vi "Get data product.vi"(8 "error in (no error)":errorcluster, 9 "Credito":dbl, 10 "Selector":dbl, 11 "Paquetes Disonibles in":refnum<class "Paquetes Disonibles.lvclass">) -> (0 "error out":errorcluster, 3 "Paquetes Disonibles out":refnum<class "Paquetes Disonibles.lvclass">)   [LabVIEW 2021, in "Paquetes Disonibles.lvlib" / "Paquetes Disonibles.lvclass"]
uses:
  Paquetes Disonibles.lvclass
  C:/Program Files (x86)/National Instruments/LabVIEW 2021/vi.lib/ActorFramework/Actor/Actor.lvclass
  Paquetes Disonibles.lvclass/Paquetes Disonibles.ctl
  <vilib>/ActorFramework/Actor/Actor.lvclass/Actor.ctl
  User Interface Messages/Get Change Msg/Get Change Msg.lvclass/Get Change Msg.ctl
  <vilib>/ActorFramework/Message Enqueuer/Message Enqueuer.lvclass/Message Enqueuer.ctl
  User Interface Messages/Get Product Msg/Get Product Msg.lvclass/Get Product Msg.ctl
  <vilib>/ActorFramework/Message Enqueuer/Enqueue.vi
  User Interface Messages/Get Change Msg/Get Change Msg.lvclass
  C:/Program Files (x86)/National Instruments/LabVIEW 2021/vi.lib/ActorFramework/Message/Message.lvclass
  User Interface Messages/Get Product Msg/Get Product Msg.lvclass
  <vilib>/ActorFramework/Message Priority Queue/Priority Enqueue.vi
  <vilib>/ActorFramework/Actor/Actor.lvclass
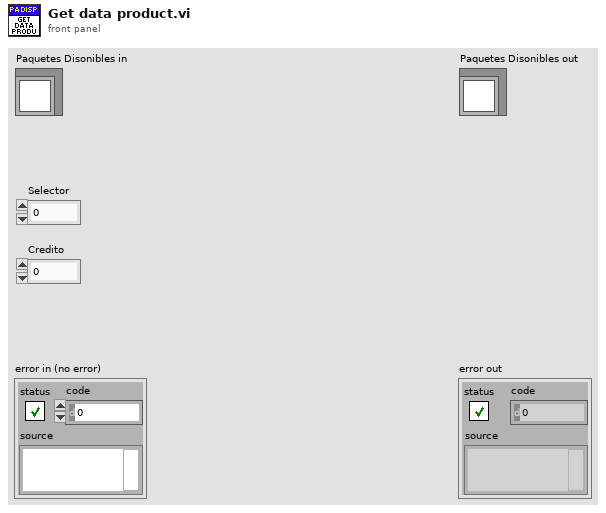
[diagram p1: front panel]
types:
  T1 = cluster{"Products":cluster{"Name":string, "Cost":u8, "Inventory":dbl}, "Products 2":cluster{"Name":string, "Cost":u8, "Inventory":dbl}, "Products 3":cluster{"Name":string, "Cost":u8, "Inventory":dbl}, "Products 4":cluster{"Name":string, "Cost":u8, "Inventory":dbl}, "Products 5":cluster{"Name":string, "Cost":u8, "Inventory":dbl}}
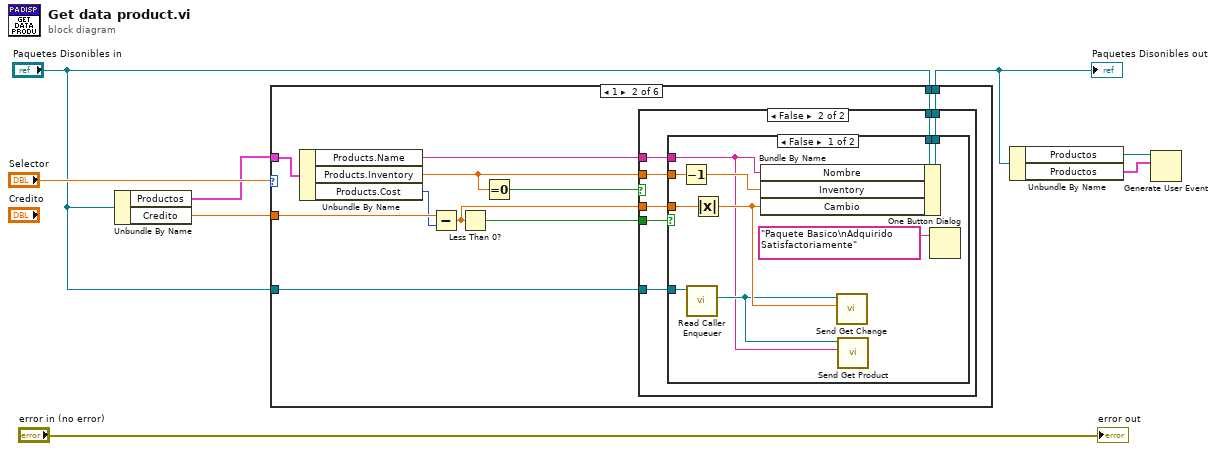
[diagram p0: block diagram]
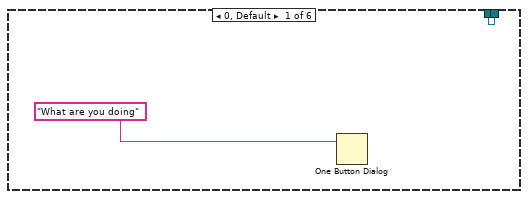
[diagram p2: hidden frame]
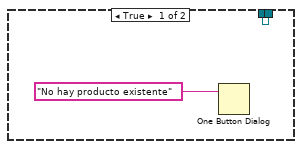
[diagram p3: hidden frame]
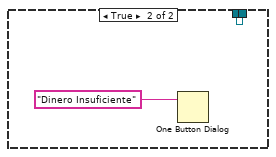
[diagram p4: hidden frame]
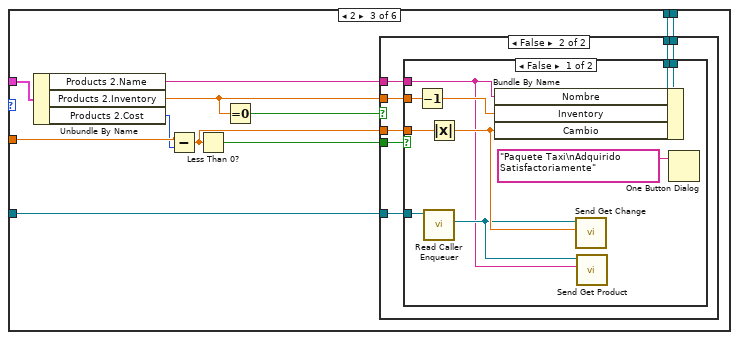
[diagram p5: hidden frame]
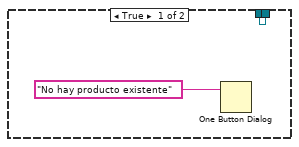
[diagram p6: hidden frame]
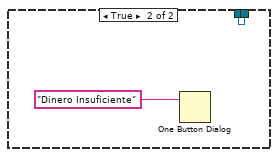
[diagram p7: hidden frame]
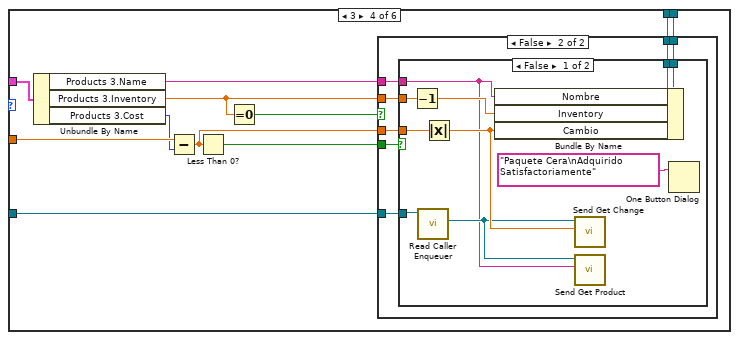
[diagram p8: hidden frame]
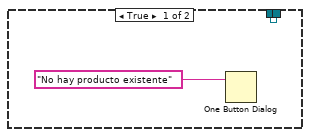
[diagram p9: hidden frame]
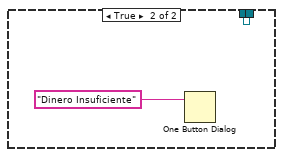
[diagram p10: hidden frame]
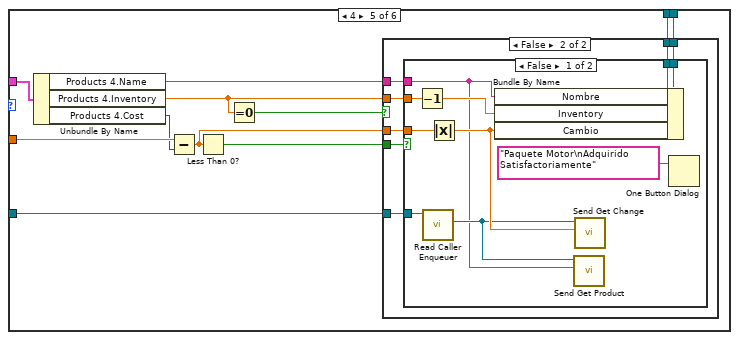
[diagram p11: hidden frame]
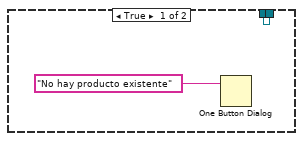
[diagram p12: hidden frame]
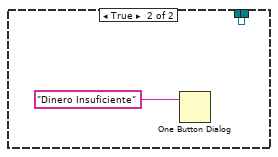
[diagram p13: hidden frame]
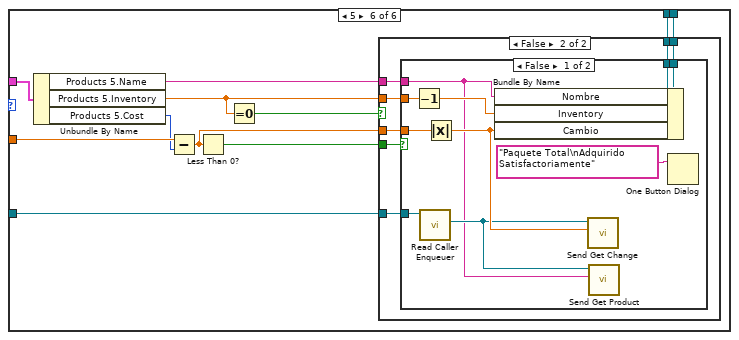
[diagram p14: hidden frame]
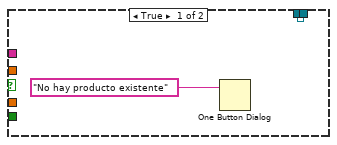
[diagram p15: hidden frame]
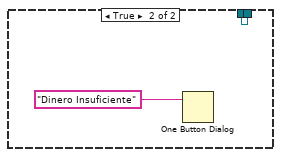
[diagram p16: hidden frame]
diagram:
  n1 = Unbundle By Name("Paquetes Disonibles in") -> ("Productos"=w6:T1, "Credito"=w2:dbl)
  n2 = case shown="1" "Selector" {
    tunnel: w2 -> [_ w15 w47 w79 w111 w143]
    tunnel: w6 -> [_ w21 w53 w85 w117 w149]
    tunnel: "Paquetes Disonibles in" -> [w10 w18 w50 w82 w114 w146]
    tunnel: [w10 w17 w49 w81 w113 w145] -> w5
    tunnel: "Paquetes Disonibles in" -> [_ w11 w43 w75 w107 w139]
    frame 0, Default {
      n3 = One Button Dialog(message="What are you doing") -> ()  [unwired: 1 in, 1 out]
    }
    frame 1 {
      n4 = Unbundle By Name(w21) -> ("Products.Name"=w19:string, "Products.Inventory"=w12:dbl, "Products.Cost"=w14:u8)
      n5 = Subtract(x=w15, y=w14) -> (x-y=w16:dbl)
      n6 = Less Than 0?(x=w16) -> (x < 0?=w20:bool)
      n7 = Equal To 0?(x=w12) -> (x = 0?=w13:bool)
      n8 = case shown="False" w13 {
        tunnel: w20 -> [_ w30]
        tunnel: w12 -> [_ w29]
        tunnel: w19 -> [_ w28]
        tunnel: w18 -> [w22 w27]
        tunnel: [w22 w26] -> w17
        tunnel: w16 -> [_ w25]
        tunnel: w11 -> [_ w24]
        frame True {
          n9 = One Button Dialog(message="No hay producto existente") -> ()  [unwired: 1 in, 1 out]
        }
        frame False {
          n10 = case shown="False" w30 {
            tunnel: w29 -> [w40 _]
            tunnel: w28 -> [w31 _]
            tunnel: w27 -> [w39 w41]
            tunnel: [w38 w41] -> w26
            tunnel: w25 -> [w36 _]
            tunnel: w24 -> [w34 _]
            frame False {
              n11 = Decrement(x=w40) -> (x-1=w37:dbl)
              n12 = call <vilib>:"Read Caller Enqueuer.vi"("Actor"=w34) -> ("Caller Enqueuer"=w32:refnum<class "Message Enqueuer.lvclass">)  [unwired: 10 in]
              n13 = Absolute Value(x=w36) -> (abs(x)=w33:dbl)
              n14 = Bundle By Name(cluster=w39, "Nombre"=w31, "Inventory"=w37, "Cambio"=w33) -> (w38:refnum<class "Paquetes Disonibles.lvclass">)
              n15 = call "Send Get Change.vi"("Cambio"=w33, "Message Enqueuer"=w32) -> ()  [unwired: 8 in, 2 out]
              n16 = call "Send Get Product.vi"("Producto"=w31, "Message Enqueuer"=w32) -> ()  [unwired: 8 in, 2 out]
              n17 = One Button Dialog(message="Paquete Basico\nAdquirido Satisfactoriamente") -> ()  [unwired: 1 in, 1 out]
            }
            frame True {
              n18 = One Button Dialog(message="Dinero Insuficiente") -> ()  [unwired: 1 in, 1 out]
            }
          }
        }
      }
    }
    frame 2 {
      n19 = Unbundle By Name(w53) -> ("Products 2.Name"=w51:string, "Products 2.Inventory"=w44:dbl, "Products 2.Cost"=w46:u8)
      n20 = Subtract(x=w47, y=w46) -> (x-y=w48:dbl)
      n21 = Less Than 0?(x=w48) -> (x < 0?=w52:bool)
      n22 = Equal To 0?(x=w44) -> (x = 0?=w45:bool)
      n23 = case shown="False" w45 {
        tunnel: w52 -> [_ w62]
        tunnel: w44 -> [_ w61]
        tunnel: w51 -> [_ w60]
        tunnel: w50 -> [w55 w59]
        tunnel: [w55 w58] -> w49
        tunnel: w48 -> [_ w57]
        tunnel: w43 -> [_ w56]
        frame True {
          n24 = One Button Dialog(message="No hay producto existente") -> ()  [unwired: 1 in, 1 out]
        }
        frame False {
          n25 = case shown="False" w62 {
            tunnel: w61 -> [w72 _]
            tunnel: w60 -> [w63 _]
            tunnel: w59 -> [w71 w73]
            tunnel: [w70 w73] -> w58
            tunnel: w57 -> [w68 _]
            tunnel: w56 -> [w66 _]
            frame False {
              n26 = Decrement(x=w72) -> (x-1=w69:dbl)
              n27 = call <vilib>:"Read Caller Enqueuer.vi"("Actor"=w66) -> ("Caller Enqueuer"=w64:refnum<class "Message Enqueuer.lvclass">)  [unwired: 10 in]
              n28 = Absolute Value(x=w68) -> (abs(x)=w65:dbl)
              n29 = Bundle By Name(cluster=w71, "Nombre"=w63, "Inventory"=w69, "Cambio"=w65) -> (w70:refnum<class "Paquetes Disonibles.lvclass">)
              n30 = call "Send Get Change.vi"("Cambio"=w65, "Message Enqueuer"=w64) -> ()  [unwired: 8 in, 2 out]
              n31 = call "Send Get Product.vi"("Producto"=w63, "Message Enqueuer"=w64) -> ()  [unwired: 8 in, 2 out]
              n32 = One Button Dialog(message="Paquete Taxi\nAdquirido Satisfactoriamente") -> ()  [unwired: 1 in, 1 out]
            }
            frame True {
              n33 = One Button Dialog(message="Dinero Insuficiente") -> ()  [unwired: 1 in, 1 out]
            }
          }
        }
      }
    }
    frame 3 {
      n34 = Unbundle By Name(w85) -> ("Products 3.Name"=w83:string, "Products 3.Inventory"=w76:dbl, "Products 3.Cost"=w78:u8)
      n35 = Subtract(x=w79, y=w78) -> (x-y=w80:dbl)
      n36 = Less Than 0?(x=w80) -> (x < 0?=w84:bool)
      n37 = Equal To 0?(x=w76) -> (x = 0?=w77:bool)
      n38 = case shown="False" w77 {
        tunnel: w84 -> [_ w94]
        tunnel: w76 -> [_ w93]
        tunnel: w83 -> [_ w92]
        tunnel: w82 -> [w87 w91]
        tunnel: [w87 w90] -> w81
        tunnel: w80 -> [_ w89]
        tunnel: w75 -> [_ w88]
        frame True {
          n39 = One Button Dialog(message="No hay producto existente") -> ()  [unwired: 1 in, 1 out]
        }
        frame False {
          n40 = case shown="False" w94 {
            tunnel: w93 -> [w104 _]
            tunnel: w92 -> [w95 _]
            tunnel: w91 -> [w103 w105]
            tunnel: [w102 w105] -> w90
            tunnel: w89 -> [w100 _]
            tunnel: w88 -> [w98 _]
            frame False {
              n41 = Decrement(x=w104) -> (x-1=w101:dbl)
              n42 = call <vilib>:"Read Caller Enqueuer.vi"("Actor"=w98) -> ("Caller Enqueuer"=w96:refnum<class "Message Enqueuer.lvclass">)  [unwired: 10 in]
              n43 = Absolute Value(x=w100) -> (abs(x)=w97:dbl)
              n44 = Bundle By Name(cluster=w103, "Nombre"=w95, "Inventory"=w101, "Cambio"=w97) -> (w102:refnum<class "Paquetes Disonibles.lvclass">)
              n45 = call "Send Get Change.vi"("Cambio"=w97, "Message Enqueuer"=w96) -> ()  [unwired: 8 in, 2 out]
              n46 = call "Send Get Product.vi"("Producto"=w95, "Message Enqueuer"=w96) -> ()  [unwired: 8 in, 2 out]
              n47 = One Button Dialog(message="Paquete Cera\nAdquirido Satisfactoriamente") -> ()  [unwired: 1 in, 1 out]
            }
            frame True {
              n48 = One Button Dialog(message="Dinero Insuficiente") -> ()  [unwired: 1 in, 1 out]
            }
          }
        }
      }
    }
    frame 4 {
      n49 = Unbundle By Name(w117) -> ("Products 4.Name"=w115:string, "Products 4.Inventory"=w108:dbl, "Products 4.Cost"=w110:u8)
      n50 = Subtract(x=w111, y=w110) -> (x-y=w112:dbl)
      n51 = Less Than 0?(x=w112) -> (x < 0?=w116:bool)
      n52 = Equal To 0?(x=w108) -> (x = 0?=w109:bool)
      n53 = case shown="False" w109 {
        tunnel: w116 -> [_ w126]
        tunnel: w108 -> [_ w125]
        tunnel: w115 -> [_ w124]
        tunnel: w114 -> [w118 w123]
        tunnel: [w118 w122] -> w113
        tunnel: w112 -> [_ w121]
        tunnel: w107 -> [_ w120]
        frame True {
          n54 = One Button Dialog(message="No hay producto existente") -> ()  [unwired: 1 in, 1 out]
        }
        frame False {
          n55 = case shown="False" w126 {
            tunnel: w125 -> [w136 _]
            tunnel: w124 -> [w127 _]
            tunnel: w123 -> [w135 w137]
            tunnel: [w134 w137] -> w122
            tunnel: w121 -> [w132 _]
            tunnel: w120 -> [w129 _]
            frame False {
              n56 = Decrement(x=w136) -> (x-1=w133:dbl)
              n57 = call <vilib>:"Read Caller Enqueuer.vi"("Actor"=w129) -> ("Caller Enqueuer"=w128:refnum<class "Message Enqueuer.lvclass">)  [unwired: 10 in]
              n58 = Absolute Value(x=w132) -> (abs(x)=w130:dbl)
              n59 = Bundle By Name(cluster=w135, "Nombre"=w127, "Inventory"=w133, "Cambio"=w130) -> (w134:refnum<class "Paquetes Disonibles.lvclass">)
              n60 = call "Send Get Product.vi"("Producto"=w127, "Message Enqueuer"=w128) -> ()  [unwired: 8 in, 2 out]
              n61 = call "Send Get Change.vi"("Cambio"=w130, "Message Enqueuer"=w128) -> ()  [unwired: 8 in, 2 out]
              n62 = One Button Dialog(message="Paquete Motor\nAdquirido Satisfactoriamente") -> ()  [unwired: 1 in, 1 out]
            }
            frame True {
              n63 = One Button Dialog(message="Dinero Insuficiente") -> ()  [unwired: 1 in, 1 out]
            }
          }
        }
      }
    }
    frame 5 {
      n64 = Unbundle By Name(w149) -> ("Products 5.Name"=w147:string, "Products 5.Inventory"=w140:dbl, "Products 5.Cost"=w142:u8)
      n65 = Subtract(x=w143, y=w142) -> (x-y=w144:dbl)
      n66 = Less Than 0?(x=w144) -> (x < 0?=w148:bool)
      n67 = Equal To 0?(x=w140) -> (x = 0?=w141:bool)
      n68 = case shown="False" w141 {
        tunnel: w148 -> [_ w158]
        tunnel: w140 -> [_ w157]
        tunnel: w147 -> [_ w156]
        tunnel: w146 -> [w150 w155]
        tunnel: [w150 w154] -> w145
        tunnel: w144 -> [_ w153]
        tunnel: w139 -> [_ w152]
        frame True {
          n69 = One Button Dialog(message="No hay producto existente") -> ()  [unwired: 1 in, 1 out]
        }
        frame False {
          n70 = case shown="False" w158 {
            tunnel: w157 -> [w168 _]
            tunnel: w156 -> [w159 _]
            tunnel: w155 -> [w167 w169]
            tunnel: [w166 w169] -> w154
            tunnel: w153 -> [w164 _]
            tunnel: w152 -> [w162 _]
            frame False {
              n71 = Decrement(x=w168) -> (x-1=w165:dbl)
              n72 = call <vilib>:"Read Caller Enqueuer.vi"("Actor"=w162) -> ("Caller Enqueuer"=w160:refnum<class "Message Enqueuer.lvclass">)  [unwired: 10 in]
              n73 = Absolute Value(x=w164) -> (abs(x)=w161:dbl)
              n74 = Bundle By Name(cluster=w167, "Nombre"=w159, "Inventory"=w165, "Cambio"=w161) -> (w166:refnum<class "Paquetes Disonibles.lvclass">)
              n75 = call "Send Get Change.vi"("Cambio"=w161, "Message Enqueuer"=w160) -> ()  [unwired: 8 in, 2 out]
              n76 = call "Send Get Product.vi"("Producto"=w159, "Message Enqueuer"=w160) -> ()  [unwired: 8 in, 2 out]
              n77 = One Button Dialog(message="Paquete Total\nAdquirido Satisfactoriamente") -> ()  [unwired: 1 in, 1 out]
            }
            frame True {
              n78 = One Button Dialog(message="Dinero Insuficiente") -> ()  [unwired: 1 in, 1 out]
            }
          }
        }
      }
    }
  }
  "Paquetes Disonibles out" <- w5
  n79 = Unbundle By Name(w5) -> ("Productos"=w4:refnum<user-event>, "Productos"=w3:T1)
  n80 = Generate User Event(user event=w4, event data cluster=w3) -> ()  [unwired: 2 in, 2 out]
  "error out" <- "error in (no error)"
